vi "Call Function.vi"() -> ()   [LabVIEW 2022 SP3, in "Python Driver.lvclass"]
uses:
  Python Driver.lvclass
panel:
  out "error out":errorcluster
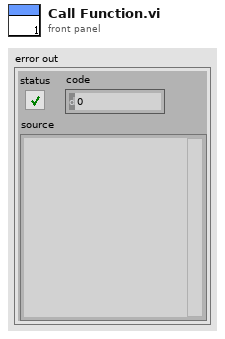
[diagram p1: front panel]
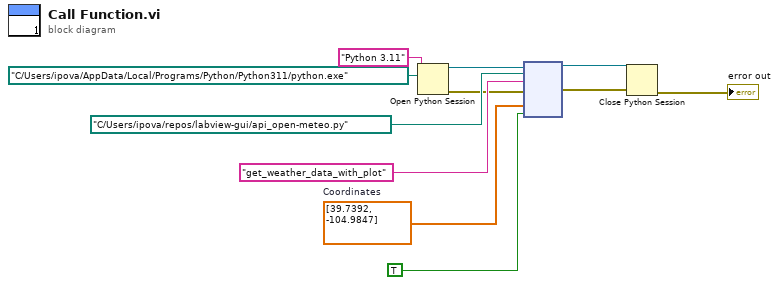
[diagram p0: block diagram]
diagram:
  w6 = dbl[] [39.7392, -104.9847]  # Coordinates
  n1 = Open Python Session(python version="Python 3.11" ("Python version"), python path=path "C:/Users/ipova/AppData/Local/Programs/Python/Python311/python.exe" ("Python path")) -> (session out=w9:refnum<k35>, error out=w5:errorcluster)  [unwired: 1 in]
  n2 = node(w9, path "C:/Users/ipova/repos/labview-gui/api_open-meteo.py" ("module path"), "get_weather_data_with_plot" ("function name"), w5, w6, TRUE) -> (w3:refnum<k35>, w2:errorcluster)  [unwired: 4 in, 2 out]
  n3 = Close Python Session(session in=w3, error in=w2) -> (11:→"error out":errorcluster)
